vi "Login.vi"() -> ()   [LabVIEW 2015]
uses:
  _typedef/userOfLoginLaw.ctl
  Management/Management_class/Display.lvclass
  <vilib>/ActorFramework/Actor/Actor.lvclass
panel:
  in  "admin":bool
  in  "commonUser":bool
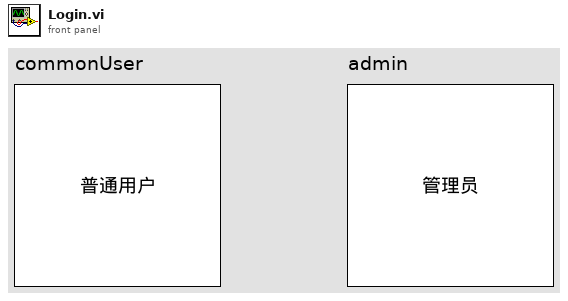
[diagram p1: front panel]
types:
  T1 = typedef "userOfLoginLaw.ctl" = enum16{"COMMONUSER", "ADMIN"}
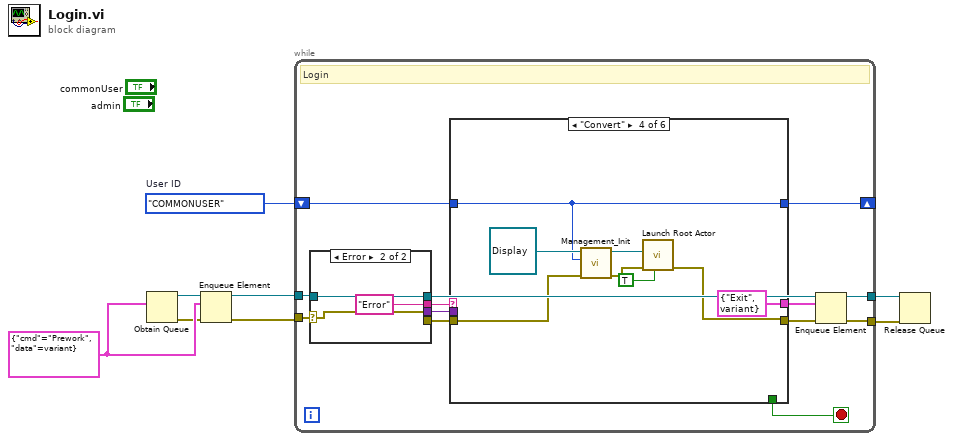
[diagram p0: block diagram]
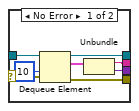
[diagram p2: hidden frame]
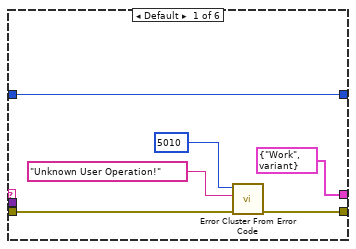
[diagram p3: hidden frame]
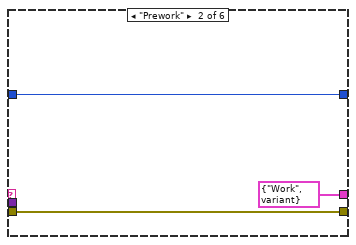
[diagram p4: hidden frame]
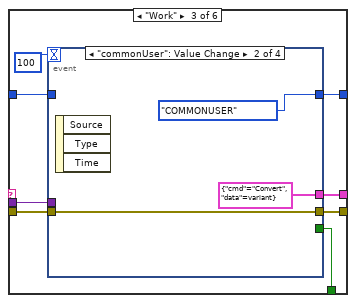
[diagram p5: hidden frame]
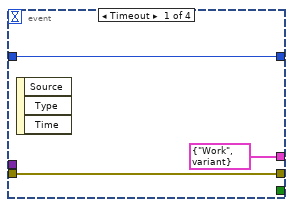
[diagram p6: hidden frame]
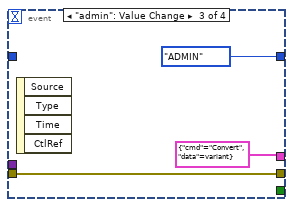
[diagram p7: hidden frame]
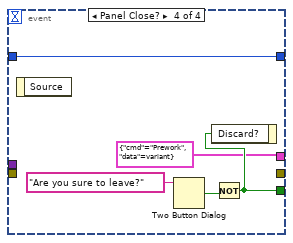
[diagram p8: hidden frame]
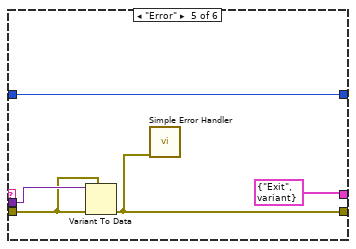
[diagram p9: hidden frame]
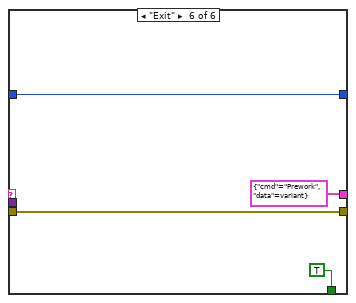
[diagram p10: hidden frame]
diagram:
  w1 = userOfLoginLaw."COMMONUSER"  # User ID
  w6 = cluster{"cmd":string, "data":variant} {"cmd"="Prework", "data"=variant}
  n1 = Obtain Queue(element data type=w6) -> (queue out=w2:refnum<queue>, error out=w3:errorcluster)  [unwired: 4 in, 1 out]
  n2 = Enqueue Element(queue=w2, element=w6, error in (no error)=w3) -> (queue out=w4:refnum<queue>, error out=w5:errorcluster)  [unwired: 1 in, 1 out]
  n3 = while {
    tunnel: w4 -> [w20]
    tunnel: w5 -> [w21]
    tunnel: [w12] -> w7
    tunnel: [w11] -> w8
    shift-right: [w9] -> _
    shift-left: w1 -> [w10]
    stop <- w13 stop-if-true
    # "Login"
    n4 = case shown="Error" w21 {
      selector: w21 -> [w28 w31]
      tunnel: w20 -> [w29 w32]
      tunnel: [w26 w32] -> w18
      tunnel: [w25 _] -> w16
      tunnel: [w23 "Error" ("cmd")] -> w17
      tunnel: [w22 w31] -> w19
      frame No Error {
        n5 = Dequeue Element(queue=w29, timeout in ms (-1)=10, error in (no error)=w28) -> (queue out=w26:refnum<queue>, element=w24:cluster{"cmd":string, "data":variant}, error out=w25:errorcluster)  [unwired: 1 out]
        n6 = Unbundle(w24) -> ("cmd"=w23:string, "data"=w22:variant)
      }
      frame Error {
      }
    }
    n7 = case shown="\"Convert\"" w17 {
      tunnel: w19 -> [_ _ w49 _ w76 _]
      tunnel: w16 -> [w35 w41 w48 w66 w75 w80]
      tunnel: [cluster{"cmd":string, "data":variant} {"cmd"="Work", "data"=variant} cluster{"cmd":string, "data":variant} {"cmd"="Work", "data"=variant} w46 cluster{"cmd":string, "data":variant} {"cmd"="Exit", "data"=variant} cluster{"cmd":string, "data":variant} {"cmd"="Exit", "data"=variant} cluster{"cmd":string, "data":variant} {"cmd"="Prework", "data"=variant}] -> w15
      tunnel: [w36 w41 w45 w65 w73 w80] -> w14
      tunnel: [_ _ w44 _ _ TRUE] -> w13
      tunnel: w10 -> [w33 w39 w43 w69 w72 w77]
      tunnel: [w33 w39 w42 w69 w72 w77] -> w9
      frame Default {
        n8 = call <vilib>:"Error Cluster From Error Code.vi"("error in (no error)"=w35, "error message (\"\")"="Unknown User Operation!" ("error message (\"\")"), "error code (0)"=5010) -> ("error out"=w36:errorcluster)  [unwired: 6 in]
      }
      frame "Prework" {
      }
      frame "Work" {
        n9 = event shown="[1] \"commonUser\": Value Change" {
          selector: _ -> [_ _ _ _]
          dyn-events: _ -> [_ _ _ _]
          timeout: 100 -> [_ _ _ _]
          tunnel: w49 -> [_ _ _ _]
          tunnel: w48 -> [w51 w53 w56 _]
          tunnel: [cluster{"cmd":string, "data":variant} {"cmd"="Work", "data"=variant} cluster{"cmd":string, "data":variant} {"cmd"="Convert", "data"=variant} cluster{"cmd":string, "data":variant} {"cmd"="Convert", "data"=variant} cluster{"cmd":string, "data":variant} {"cmd"="Prework", "data"=variant}] -> w46
          tunnel: [w51 w53 w56 _] -> w45
          tunnel: [_ _ _ w61] -> w44
          tunnel: w43 -> [w50 _ _ w60]
          tunnel: [w50 userOfLoginLaw."COMMONUSER" ("LAW") userOfLoginLaw."ADMIN" ("LAW") w60] -> w42
          event Timeout {
            n10 = event-data() -> ()  [unwired: 1 in, 3 out]
          }
          event "commonUser": Value Change {
            n11 = event-data() -> ()  [unwired: 1 in, 3 out]
          }
          event "admin": Value Change {
            n12 = event-data() -> ()  [unwired: 1 in, 4 out]
          }
          event Panel Close? {
            n13 = event-data() -> ()  [unwired: 1 in, 1 out]
            n14 = Two Button Dialog(message="Are you sure to leave?") -> (T button?=w62:bool)  [unwired: 2 in]
            n15 = Not(x=w62) -> (.not. x?=w61:bool)
            n16 = event-data("Discard?"=w61) -> ()  [unwired: 1 in, 1 out]
          }
        }
      }
      frame "Convert" {
        n17 = call "Management_Init.vi"("error in (no error)"=w66, "LAW"=w69, "object in"=refnum<class "Display.lvclass"> refnum) -> ("error out"=w67:errorcluster, "object out"=w68:refnum<class "Display.lvclass">)  [unwired: 6 in]
        n18 = call <vilib>:"Launch Root Actor.vi"("Open Actor Core front panel? (F)"=TRUE, "error in (no error)"=w67, "Actor"=w68) -> ("error out"=w65:errorcluster)  [unwired: 7 in, 1 out]
      }
      frame "Error" {
        n19 = Variant To Data(error in=w75, type=w75, Variant=w76) -> (error out=w73:errorcluster)  [unwired: 1 out]
        n20 = call <vilib>:"Simple Error Handler.vi"("error in (no error)"=w73) -> ()  [unwired: 4 in, 5 out]
      }
      frame "Exit" {
      }
    }
    n21 = Enqueue Element(queue=w18, element=w15, error in (no error)=w14) -> (queue out=w12:refnum<queue>, error out=w11:errorcluster)  [unwired: 1 in, 1 out]
  }
  n22 = Release Queue(queue=w7, error in (no error)=w8) -> ()  [unwired: 1 in, 3 out]
